vi "Apply Trapezoid.vi"(6 "FeedForward Constants":cluster{"kA":dbl, "kS":dbl, "kG":dbl, "kV":dbl}, 9 "Velocity values":dbl[](array[numeric]), 10 "MotorControlDeviceRef in":T1) -> (1 "Sensor Position":dbl, 2 "MotorControlDevRef out":T1, 3 "Boolean":bool, 4 "charted V":cluster{"Sensor Velocity":dbl, "Numeric":dbl}[](array[cluster]))   [LabVIEW 2023]
uses:
  <vilib>/Rock Robotics/WPI/MotorControl/WPI_MotorControlDeviceRef.ctl
  <vilib>/Rock Robotics/WPI/MotorControl/WPI_MotorControlType.ctl
  <vilib>/Rock Robotics/SystemInterfaces/DIO/FPGA_DIOPWMChannel.ctl
  <vilib>/Rock Robotics/WPI/PWM/WPI_PWMDeadband.ctl
  <vilib>/Rock Robotics/SystemInterfaces/DIO/FPGA_DIOChannel.ctl
  <vilib>/Platform/TimedLoop/XDataNode/timing_clust.ctl
  <vilib>/Platform/TimedLoop/XDataNode/nitl_modes.ctl
  <vilib>/Platform/TimedLoop/XDataNode/wakeup.ctl
  <vilib>/Rock Robotics/WPI/ThirdParty/REV Robotics/REVLib/Typedef/Spark MAX Control Type.ctl
  <vilib>/Rock Robotics/WPI/ThirdParty/REV Robotics/REVLib/Typedef/SPARK Closed Loop Slot.ctl
  <vilib>/Rock Robotics/WPI/ThirdParty/REV Robotics/REVLib/SubVI/Public/SPARK Get Encoder Status Velocity.vi
  <vilib>/Rock Robotics/WPI/ThirdParty/REV Robotics/REVLib/SubVI/Public/SPARK Get Encoder Status Position.vi
  <vilib>/Platform/TimedLoop/XDataNode/XDataNode.xnode
  <vilib>/Platform/TimedLoop/XDataNode/XDNodeRunTimeDep.lvlib
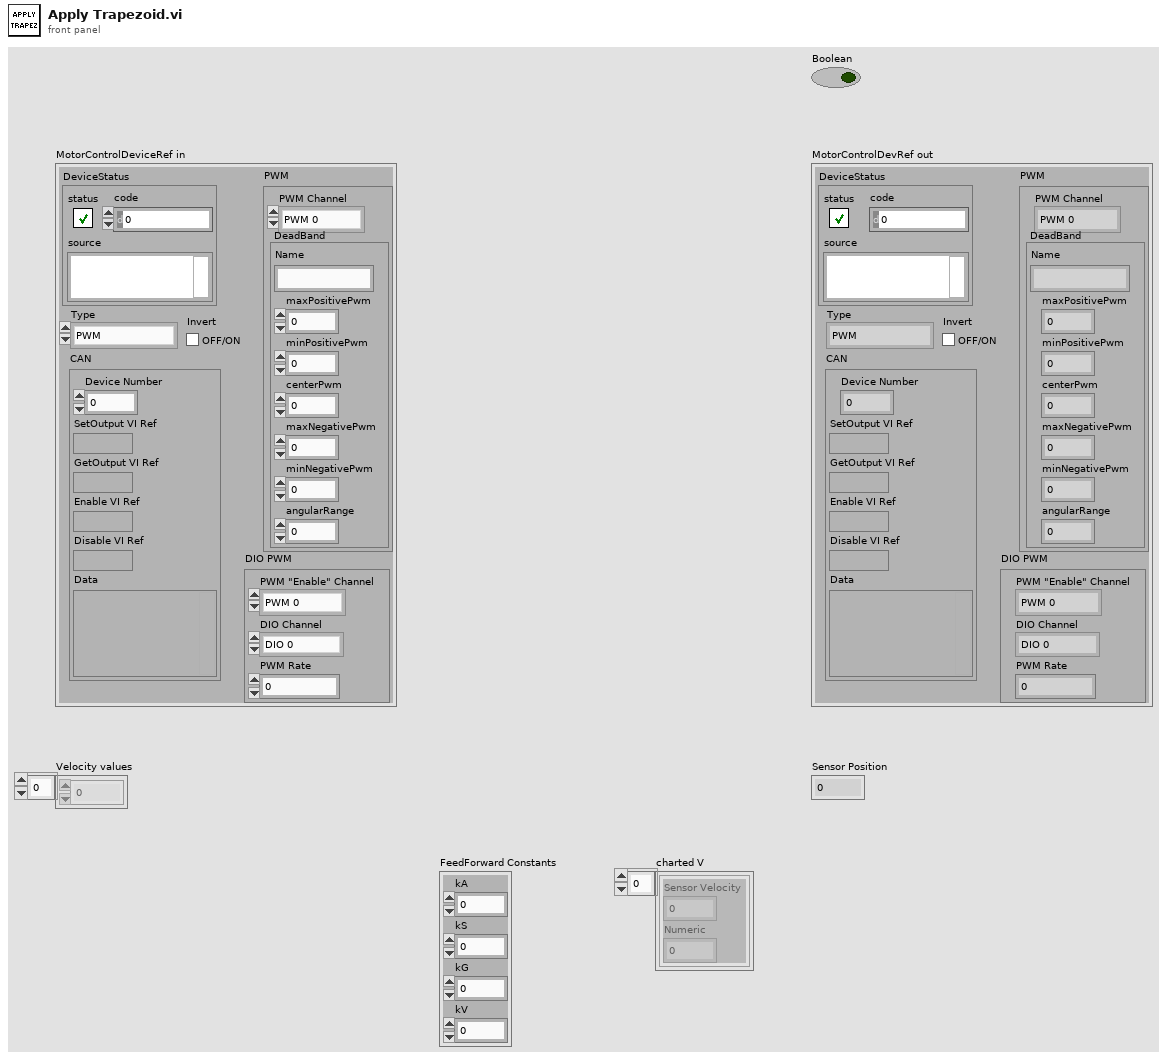
[diagram p1: front panel]
types:
  T1 = typedef "WPI_MotorControlDeviceRef.ctl" = cluster{"DeviceStatus":errorcluster, "Type":T2, "PWM":cluster{"PWM Channel":T3, "DeadBand":T4}, "CAN":cluster{"Device Number":u8, "SetOutput VI Ref":variant, "GetOutput VI Ref":variant, "Enable VI Ref":variant, "Disable VI Ref":variant, "Data":variant}, "Invert":bool, "DIO PWM":cluster{"PWM \"Enable\" Channel":T3, "DIOChannel":T5, "PWM Rate":dbl}}
  T2 = typedef "WPI_MotorControlType.ctl" = enum16{"PWM", "CAN", "DIO PWM"}
  T3 = typedef "FPGA_DIOPWMChannel.ctl" = enum8{"PWM 0", "PWM 1", "PWM 2", "PWM 3", "PWM 4", "PWM 5", "PWM 6", "PWM 7", "PWM 8", "PWM 9", "PWM MXP 0", "PWM MXP 1", "PWM MXP 2", "PWM MXP 3", "PWM MXP 4", "PWM MXP 5", "PWM MXP 6", "PWM MXP 7", "PWM MXP 8", "PWM MXP 9", "Invalid"}
  T4 = typedef "WPI_PWMDeadband.ctl" = cluster{"Name":string, "maxPositivePwm":i32, "minPositivePwm":i32, "centerPwm":i32, "maxNegativePwm":i32, "minNegativePwm":i32, "angularRange":u16}
  T5 = typedef "FPGA_DIOChannel.ctl" = enum8{"DIO 0", "DIO 1", "DIO 2", "DIO 3", "DIO 4", "DIO 5", "DIO 6", "DIO 7", "DIO 8", "DIO 9", "DIO MXP 0", "DIO MXP 1", "DIO MXP 2", "DIO MXP 3", "DIO MXP 4", "DIO MXP 5", "DIO MXP 6", "DIO MXP 7", "DIO MXP 8", "DIO MXP 9", "DIO MXP 10", "DIO MXP 11", "DIO MXP 12", "DIO MXP 13", "DIO MXP 14", "DIO MXP 15", "SPI Port CS1", "SPI Port CS2", "SPI Port CS3", "SPI Port MISO", "SPI Port MOSI", "Invalid"}
  T6 = typedef "XDNodeRunTimeDep.lvlib/timing_clust.ctl" = cluster{"Expected End [f-1]":u64, "Actual End [f-1]":u64, "Finished Late? [f-1]":bool, "Expected End [i-1]":u64, "Actual End [i-1]":u64, "Finished Late? [i-1]":bool, "Expected Start [i]":u64, "Actual Start [i]":u64, "Expected Start [f]":u64, "Actual Start [f]":u64, "Source Name":string, "Structure Name":string, "Period":i64, "Deadline":i64, "Offset":i64, "Start":i64, "Priority":i32, "Timeout":i32, "Mode":T7, "Wakeup Reason":T8, "Error":errorcluster, "Source Type":string, "Secondary Source Type":string, "Global End Time":u64, "Global Start Time":u64, "Frame Duration":u64, "Iteration Duration":u64, "Assigned CPU":i32, "I/O Scan Engine Mode":u32}
  T7 = typedef "XDNodeRunTimeDep.lvlib/nitl_modes.ctl" = enum32{"No Change", "Process missed periods, maintain original phase", "Discard missed periods, maintain original phase", "Process missed periods, ignore original phase", "Discard missed periods, ignore original phase"}
  T8 = typedef "XDNodeRunTimeDep.lvlib/wakeup.ctl" = enum32{"Normal", "Aborted", "Asynchronous wakeup", "Timing source error", "Timed loop error", "Timeout"}
  T9 = typedef "Spark MAX Control Type.ctl" = enum16{"Percent VBus", "Voltage", "Velocity", "Position", "Smart Motion", "Current", "Smart Velocity", "MAXMotion Position", "MAXMotion Velocity"}
  T10 = typedef "SPARK Closed Loop Slot.ctl" = u16
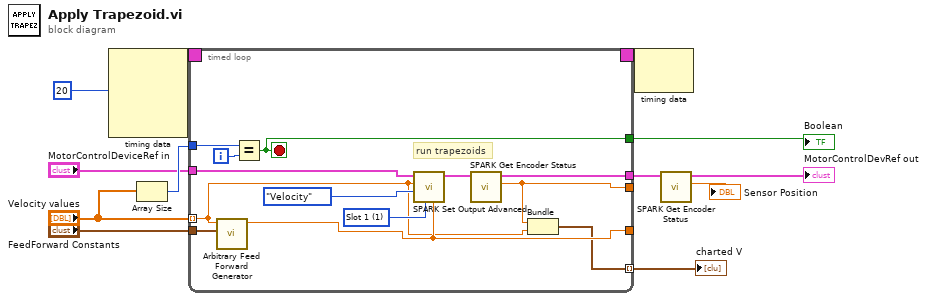
[diagram p0: block diagram]
diagram:
  n1 = node-c288(i64 20 ("Period")) -> (w12:T6)  [unwired: 3 in]
  n2 = Array Size(array="Velocity values") -> (size(s)=w8:i32)
  n3 = timed-loop {
    timing: w12 -> [_]
    timing-out: [_] -> w11
    tunnel: "MotorControlDeviceRef in" -> [w25]
    tunnel: w8 -> [w20]
    tunnel: [w22] -> w2
    tunnel: [w18] -> w5
    tunnel: "FeedForward Constants" -> [w19]
    tunnel: "Velocity values" -> [w14] mode=indexing
    tunnel: [w15] -> _
    tunnel: [w17] -> _
    tunnel: [w13] -> w10 mode=indexing
    i -> [w23]
    stop <- w22 stop-if-true
    w16 = T10 1 items=["Slot 0", "Slot 1", "Slot 2", "Slot 3"] ("Closed Loop Slot")
    # "run trapezoids"
    n4 = call "Arbitrary Feed Forward Generator.vi"("Feed Forward Constants"=w19, "Setpoint"=w14) -> ("Arbitrary Feedforward"=w17:dbl)  [unwired: 9 in]
    n5 = Equal?(x=w20, y=w23) -> (x = y?=w22:bool)
    n6 = call <vilib>:"SPARK Set Output Advanced.vi"("Arbitrary Feed Forward (0)"=w17, "Closed Loop Slot"=w16, "Control Mode"=Spark_MAX_Control_Type."Velocity", "Setpoint"=w14, "MotorControlDevRef"=w25) -> ("MotorControlDevRef"=w21:T1)  [unwired: 5 in, 1 out]
    n7 = call-poly <vilib>:"SPARK Get Encoder Status.vi"("MotorControlDevRef in"=w21) -> ("Sensor Velocity"=w15:dbl, "MotorControlDevRef out"=w18:T1)  [unwired: 7 in, 2 out]
    n8 = Bundle("Sensor Velocity"=w15, "Numeric"=w14) -> (w13:cluster{"Sensor Velocity":dbl, "Numeric":dbl})  [unwired: 1 in]
  }
  "charted V" <- w10
  "Boolean" <- w2
  n9 = node-c288(w11) -> ()  [unwired: 1 out]
  n10 = call-poly <vilib>:"SPARK Get Encoder Status.vi"("MotorControlDevRef in"=w5) -> ("Sensor Position"=→"Sensor Position":dbl, "MotorControlDevRef out"=→"MotorControlDevRef out":T1)  [unwired: 7 in, 2 out]
